vi "Test-Hydrodynamics method_YCC.vi"() -> ()   [LabVIEW 2014]
uses:
  <vilib>/Utility/file.llb/Read From Spreadsheet File (DBL).vi
  <vilib>/gmath/NumericalOptimization/Nonlinear Curve Fit LM formula string.vi
  <vilib>/gmath/NI_Gmath.lvlib
panel:
  out "XY Graph":cluster{dbl[], "best nonlinear fit":dbl[]}[](graph)
  out "x/y":dbl
  in  "Conversion factor (V/um)":dbl
  out "dx (V)":dbl
  out "dx2":dbl
  out "dx1":dbl
  out "Upper QPD":dbl
  out "Lower QPD":dbl
  out "Center QPD":dbl
  out "best nonlinear fit":dbl[](array[numeric])
  out "Histogram: h(x)":i32[](array[numeric])
  out "X Values":dbl[](array[numeric])
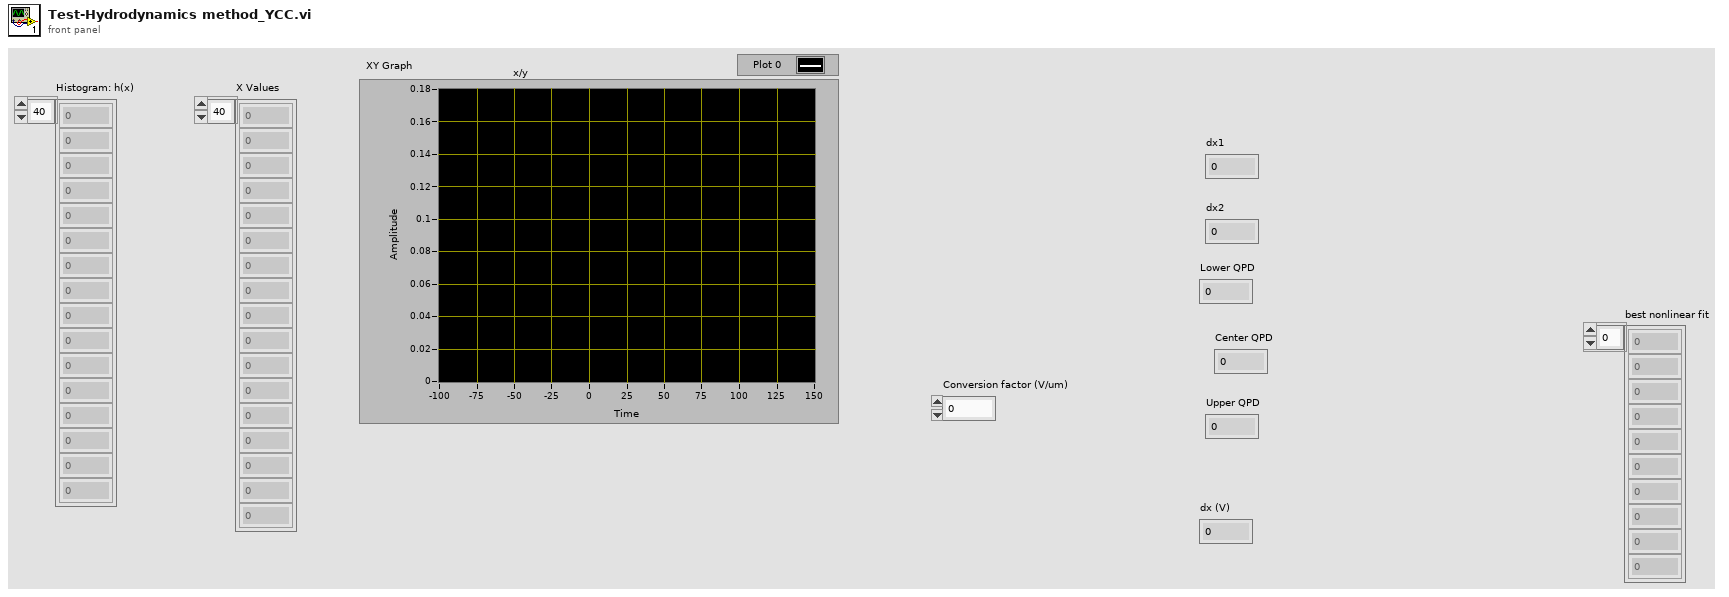
[diagram p1: front panel]
types:
  T1 = cluster{"model":string, "Parameters":string[], "x":string}
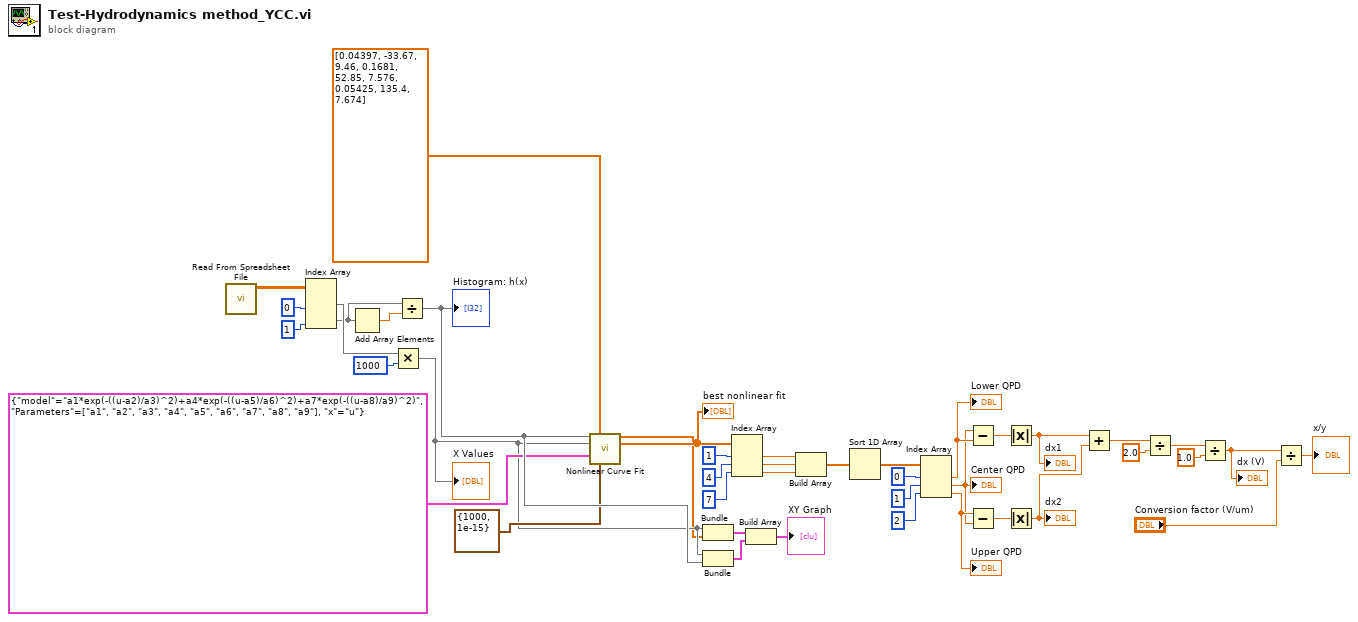
[diagram p0: block diagram]
diagram:
  n1 = call-poly <vilib>:"Read From Spreadsheet File.vi"() -> ("all rows"=w42:dbl[][])  [unwired: 7 in, 4 out]
  n2 = Index Array(array=w42, index (col) #1=0 ("disabled index (col)"), index (col) #2=1 ("index (col)")) -> (element #1=w39:dbl[], element #2=w12:dbl[])  [unwired: 2 in]
  n3 = Add Array Elements(numeric array=w12) -> (sum=w11:dbl)
  n4 = Multiply(x=w39, y=1000) -> (x*y=w7:dbl[])
  "X Values" <- w7
  n5 = Divide(x=w12, y=w11) -> (x/y=w10:dbl[])
  "Histogram: h(x)" <- w10
  n6 = call-poly <vilib>:"Nonlinear Curve Fit.vi"("Y"=w10, "initial parameters"=dbl[] [0.04397, -33.67, 9.46, 0.1681, 52.85, 7.576, 0.05425, 135.4, 7.674], "X"=w7, "model description"=T1 {"model"="a1*exp(-((u-a2)/a3)^2)+a4*exp(-((u-a5)/a6)^2)+a7*exp(-((u-a8)/a9)^2)", "Parameters"=["a1", "a2", "a3", "a4", "a5", "a6", "a7", "a8", "a9"], "x"="u"}, "termination"=cluster{"max iteration":i32, "tolerance":dbl} {"max iteration"=1000, "tolerance"=1e-15}) -> ("best nonlinear fit"=w5:dbl[], "best fit parameters"=w6:dbl[])  [unwired: 6 in, 3 out]
  "best nonlinear fit" <- w6
  n7 = Bundle(w7, "best nonlinear fit"=w5) -> (w4:cluster{dbl[], "best nonlinear fit":dbl[]})  [unwired: 1 in]
  n8 = Bundle(w7, w10) -> (w3:cluster{dbl[], dbl[]})  [unwired: 1 in]
  n9 = Index Array(array=w6, index #1=1 ("index"), index #2=4 ("index"), index #3=7 ("index")) -> (element #1=w34:dbl, element #2=w33:dbl, element #3=w32:dbl)
  n10 = Build Array(w4, w3) -> (→"XY Graph":cluster{dbl[], "best nonlinear fit":dbl[]}[])
  n11 = Build Array(w34, w33, w32) -> (w31:dbl[])
  n12 = Sort 1D Array(array=w31) -> (sorted array=w30:dbl[])
  n13 = Index Array(array=w30, index #1=0 ("index"), index #2=1 ("index"), index #3=2 ("index")) -> (element #1=w26:dbl, element #2=w24:dbl, element #3=w25:dbl)
  "Center QPD" <- w24
  "Lower QPD" <- w26
  "Upper QPD" <- w25
  n14 = Subtract(x=w24, y=w26) -> (x-y=w23:dbl)
  n15 = Subtract(x=w25, y=w24) -> (x-y=w22:dbl)
  n16 = Absolute Value(x=w23) -> (abs(x)=w21:dbl)
  "dx1" <- w21
  n17 = Absolute Value(x=w22) -> (abs(x)=w20:dbl)
  "dx2" <- w20
  n18 = Add(x=w21, y=w20) -> (x+y=w19:dbl)
  n19 = Divide(x=w19, y=2.0) -> (x/y=w16:dbl)
  n20 = Divide(x=w16, y=1.0) -> (x/y=w14:dbl)
  "dx (V)" <- w14
  n21 = Divide(x=w14, y="Conversion factor (V/um)") -> (x/y=→"x/y":dbl)
